vi "CmdGetIdentification.vi"(0 "CmdLib In":refnum<k24>, 5 "Device Key In":string, 11 "error in (no error)":errorcluster) -> (4 "CmdLib Out":refnum<k24>, 6 "Device Key Out":string, 8 "IOStatus":i32, 10 "Identification":string, 15 "error out":errorcluster)   [LabVIEW 2009]
uses:
  C:/Code/Apps/Utilities/PM2935/PMWinApp/PM_Installer/Master/Samples/1918 - 2936 Family/LabVIEW/LabVIEW 2009/PowerMeterCommands.dll
  C:/Code/Apps/Utilities/PM2935/PMWinApp/PM_Installer/Master/Samples/1918 - 2936 Family/LabVIEW/LabVIEW 2009/UsbDllWrap.dll
panel:
  in  "identification":string
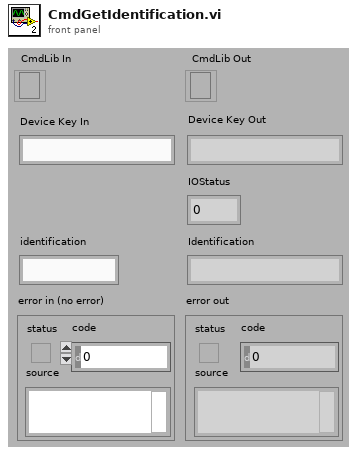
[diagram p1: front panel]
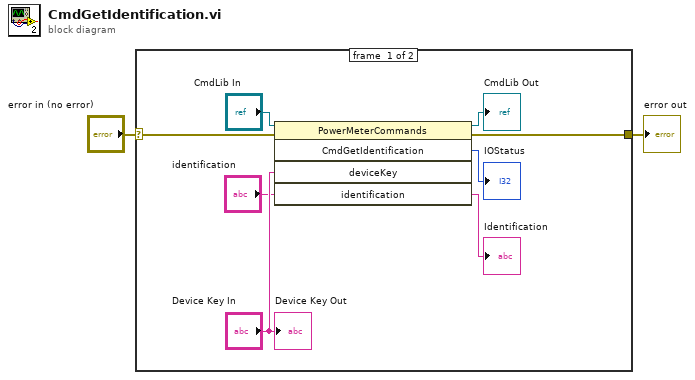
[diagram p0: block diagram]
diagram:
  n1 = case shown="No Error" "error in (no error)" {
    selector: "error in (no error)" -> [w8 w11]
    tunnel: [w10 w11] -> w1
    frame #0 {
      n2 = invoke class="PowerMeterCommands" method="CmdGetIdentification"(reference="CmdLib In", error in=w8, "deviceKey"="Device Key In", "identification"="identification") -> (reference out=→"CmdLib Out":refnum<k24>, error out=w10:errorcluster, "CmdGetIdentification"=→"IOStatus":i32, "identification"=→"Identification":string)  [unwired: 1 in, 1 out]
      "Device Key Out" <- "Device Key In"
    }
    frame #1 {
    }
  }
  "error out" <- w1
